vi "Format Symbol Name.vi"(4 "Symbol Name in":string) -> (1 "Symbol Name out":string)   [LabVIEW 2018, in "TwinCAT ADS.lvclass"]
uses:
  TwinCAT ADS.lvclass
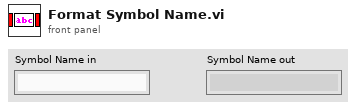
[diagram p1: front panel]
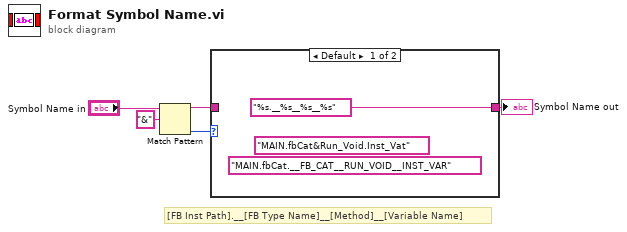
[diagram p0: block diagram]
diagram:
  # "[FB Inst Path].__[FB Type Name]__[Method]__[Variable Name]"
  n1 = Match Pattern(string="Symbol Name in", regular expression="&") -> (before substring=w2:string, offset past match=w3:i32)  [unwired: 1 in, 2 out]
  n2 = case shown="Default" w3 {
    tunnel: w2 -> [_ w7]
    tunnel: ["%s.__%s__%s__%s" ("Parent Name") w7] -> w1
    frame Default {
      (unwired) "MAIN.fbCat&Run_Void.Inst_Vat" ("Parent Name")
      (unwired) "MAIN.fbCat.__FB_CAT__RUN_VOID__INST_VAR" ("Name")
    }
    frame -1 {
    }
  }
  "Symbol Name out" <- w1
